vi "Untitled 1.vi"() -> ()   [LabVIEW 2018]
panel:
  in  "Stop 2":bool
  out "Waveform Chart":cluster{dbl, dbl}(graph)
  out "Indicator":string
  out "Temperature light":bool
  in  "Exit":bool
  in  "Settings":bool
  in  "Stop":bool
  in  "Start":bool
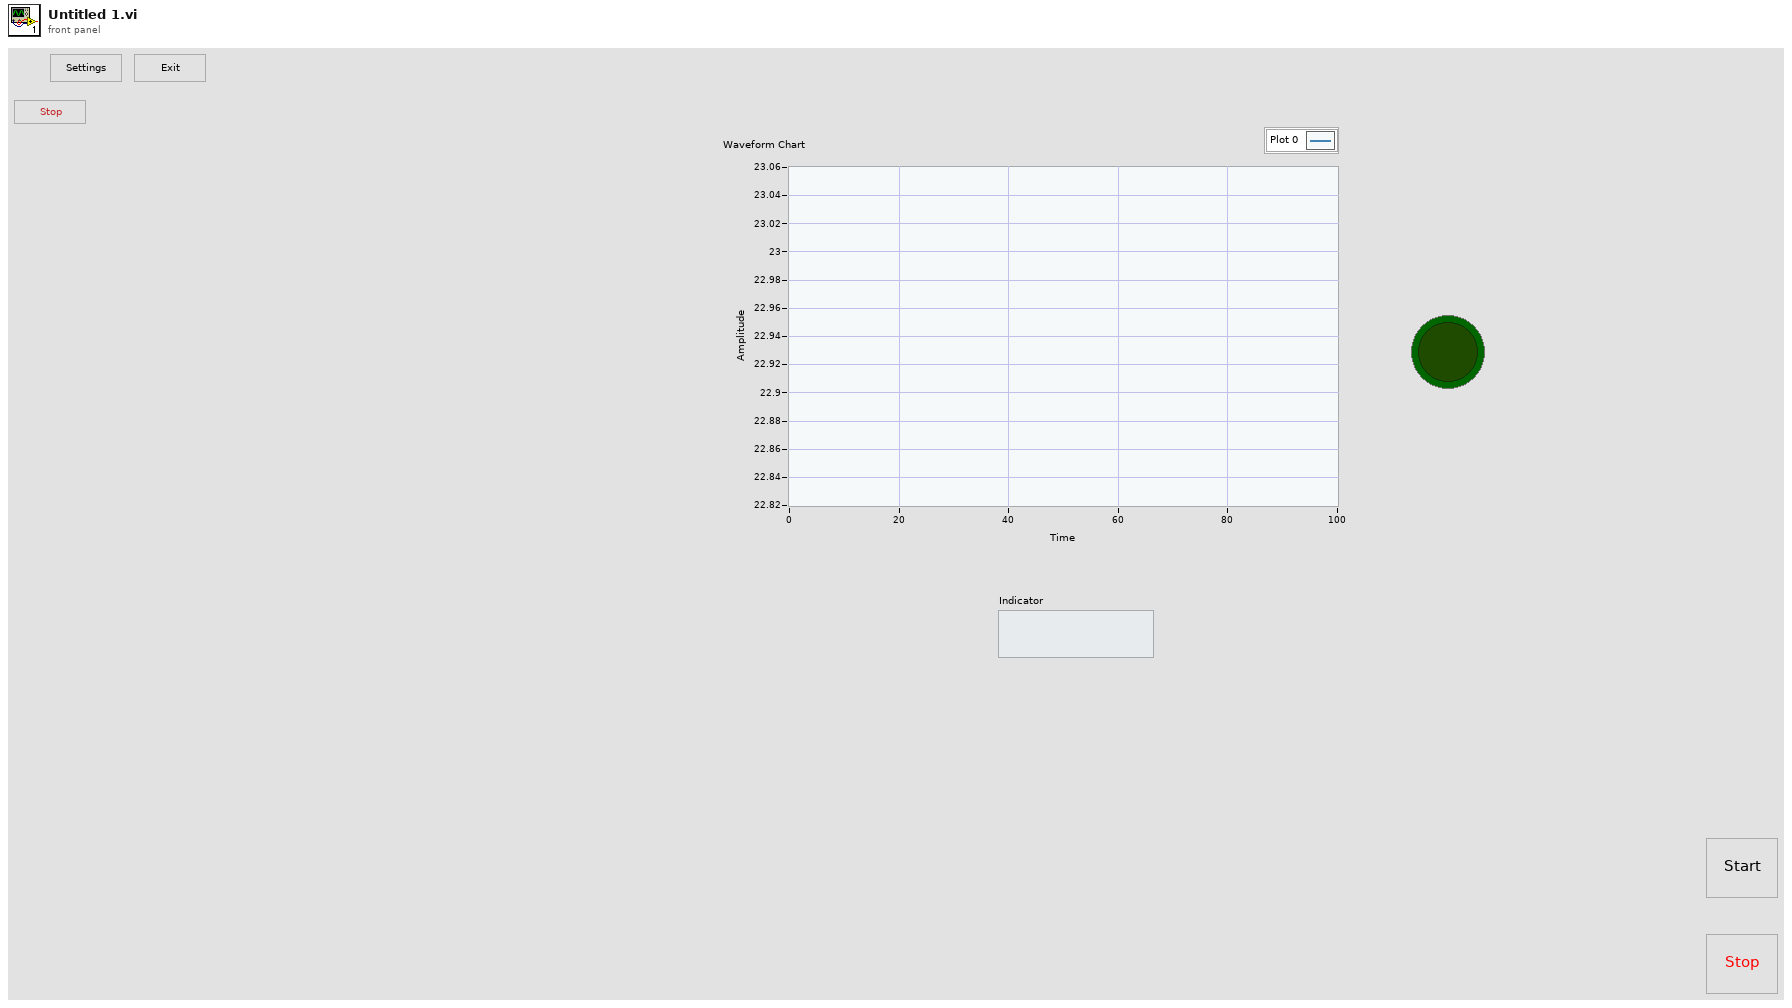
[diagram p1: front panel]
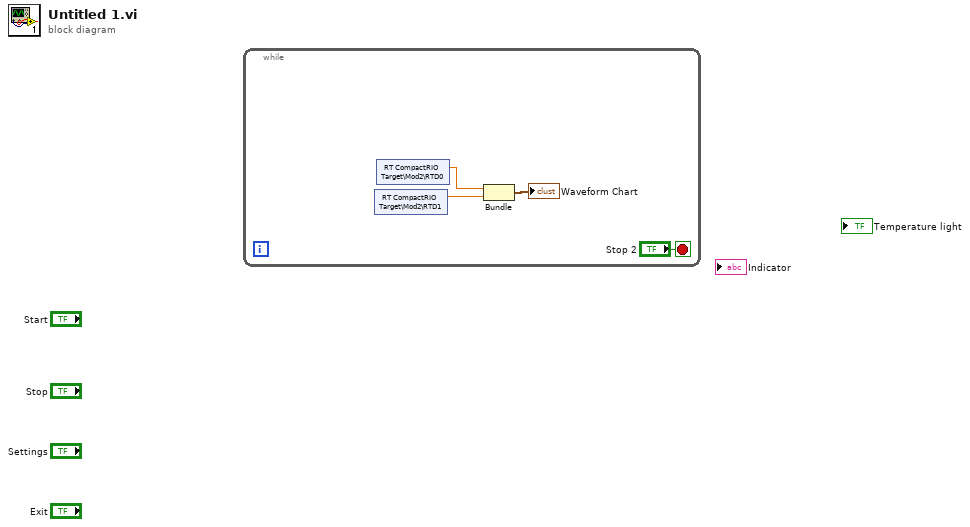
[diagram p0: block diagram]
diagram:
  n1 = while {
    stop <- "Stop 2" stop-if-true
    n2 = shared-variable "RT CompactRIO Target\\Mod2\\RTD1"() -> (w2:dbl)  [unwired: 1 in, 1 out]
    n3 = shared-variable "RT CompactRIO Target\\Mod2\\RTD0"() -> (w3:dbl)  [unwired: 1 in, 1 out]
    n4 = Bundle(w3, w2) -> (→"Waveform Chart":cluster{dbl, dbl})  [unwired: 1 in]
  }
